vi "Process.vi"(8 "Error In":errorcluster, 11 "IResult In":refnum<class "IResult.lvclass">) -> (0 "Error Out":errorcluster, 3 "IResult Out":refnum<class "IResult.lvclass">)   [LabVIEW 2020, in "IResult.lvclass"]
uses:
  IResult.lvclass
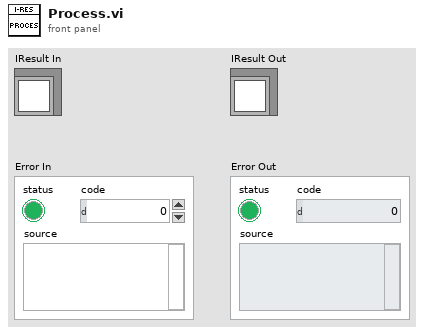
[diagram p1: front panel]
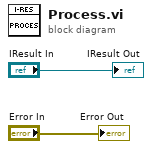
[diagram p0: block diagram]
diagram:
  "IResult Out" <- "IResult In"
  "Error Out" <- "Error In"
